vi "IMAQ Preview the image.vi"() -> ()   [LabVIEW 2018]
uses:
  LabViewDVPCamera/LabViewDVPCamera.lvlib
panel:
  in  "Video image quality (AVI format)":string
  in  "Recording Name (Path)":string
  in  "Turn on recording":bool
  out "Capture frame rate":sgl
  out "Total frame rate":u32
  out "pFrameCount out":T1
  out "frame rate":dbl format="%#.5g"
  out "value":u64
  out "Millisecond timing value 3":u32
  out "Image":T2(plugin-control)
  in  "CloseFlg":i32
  out "handle":u32
  in  "CameraList":u16(ring) items=["MGS130-H2-192.168.10.39", "MGS130-H2-192.168.10.4", "MGS203MP-H2-192.168.10.254", "MGS203MP-H2-192.168.20.2", "MGS230_YUV-H2-192.168.10.62"]
  in  "Set":bool
  in  "Close":bool
  in  "Open":bool
  in  "ScanCamera":bool
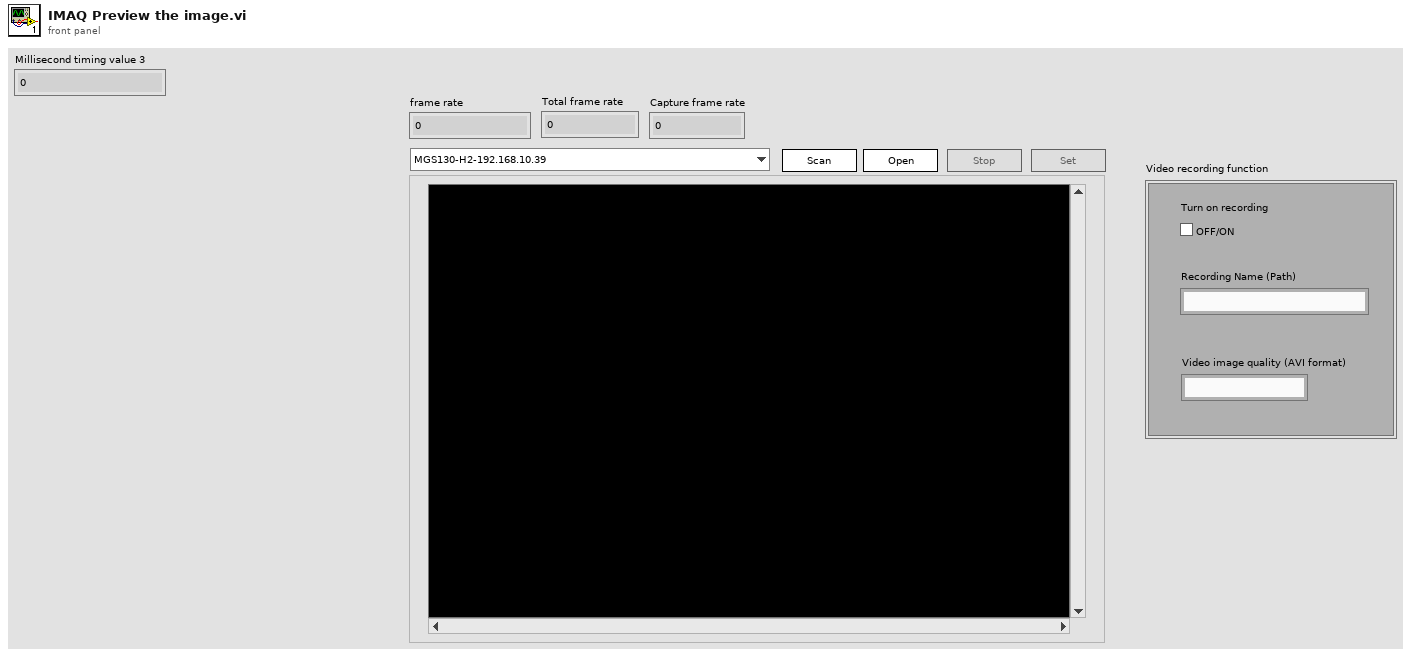
[diagram p1: front panel]
types:
  T1 = cluster{"uFrameCount":u32, "uFrameDrop":u32, "uFrameIgnore":u32, "uFrameError":u32, "uFrameOK":u32, "uFrameOut":u32, "uFrameResend":u32, "uFrameProc":u32, "fFrameRate":sgl, "fProcRate":sgl, "reserved[0]":i32, "reserved[1]":i32, "reserved[2]":i32, "reserved[3]":i32, "reserved[4]":i32, "reserved[5]":i32, "reserved[6]":i32, "reserved[7]":i32, "reserved[8]":i32, "reserved[9]":i32, "reserved[10]":i32, "reserved[11]":i32, "reserved[12]":i32, "reserved[13]":i32, "reserved[14]":i32, "reserved[15]":i32, "reserved[16]":i32, "reserved[17]":i32, "reserved[18]":i32, "reserved[19]":i32, "reserved[20]":i32, "reserved[21]":i32, "reserved[22]":i32, "reserved[23]":i32, "reserved[24]":i32, "reserved[25]":i32, "reserved[26]":i32, "reserved[27]":i32, "reserved[28]":i32, "reserved[29]":i32, "reserved[30]":i32, "reserved[31]":i32}
  T2 = typedef "IMAQ Image.ctl" = refnum<image>
  T3 = enum8{"Enabled", "Disabled", "Disabled and Grayed Out"}
  T4 = typedef "LVStringsAndValuesArrayTypeDef_U16.ctl" = cluster{"String":string, "Value":u16}[]
  T5 = typedef "Image Type" = u32
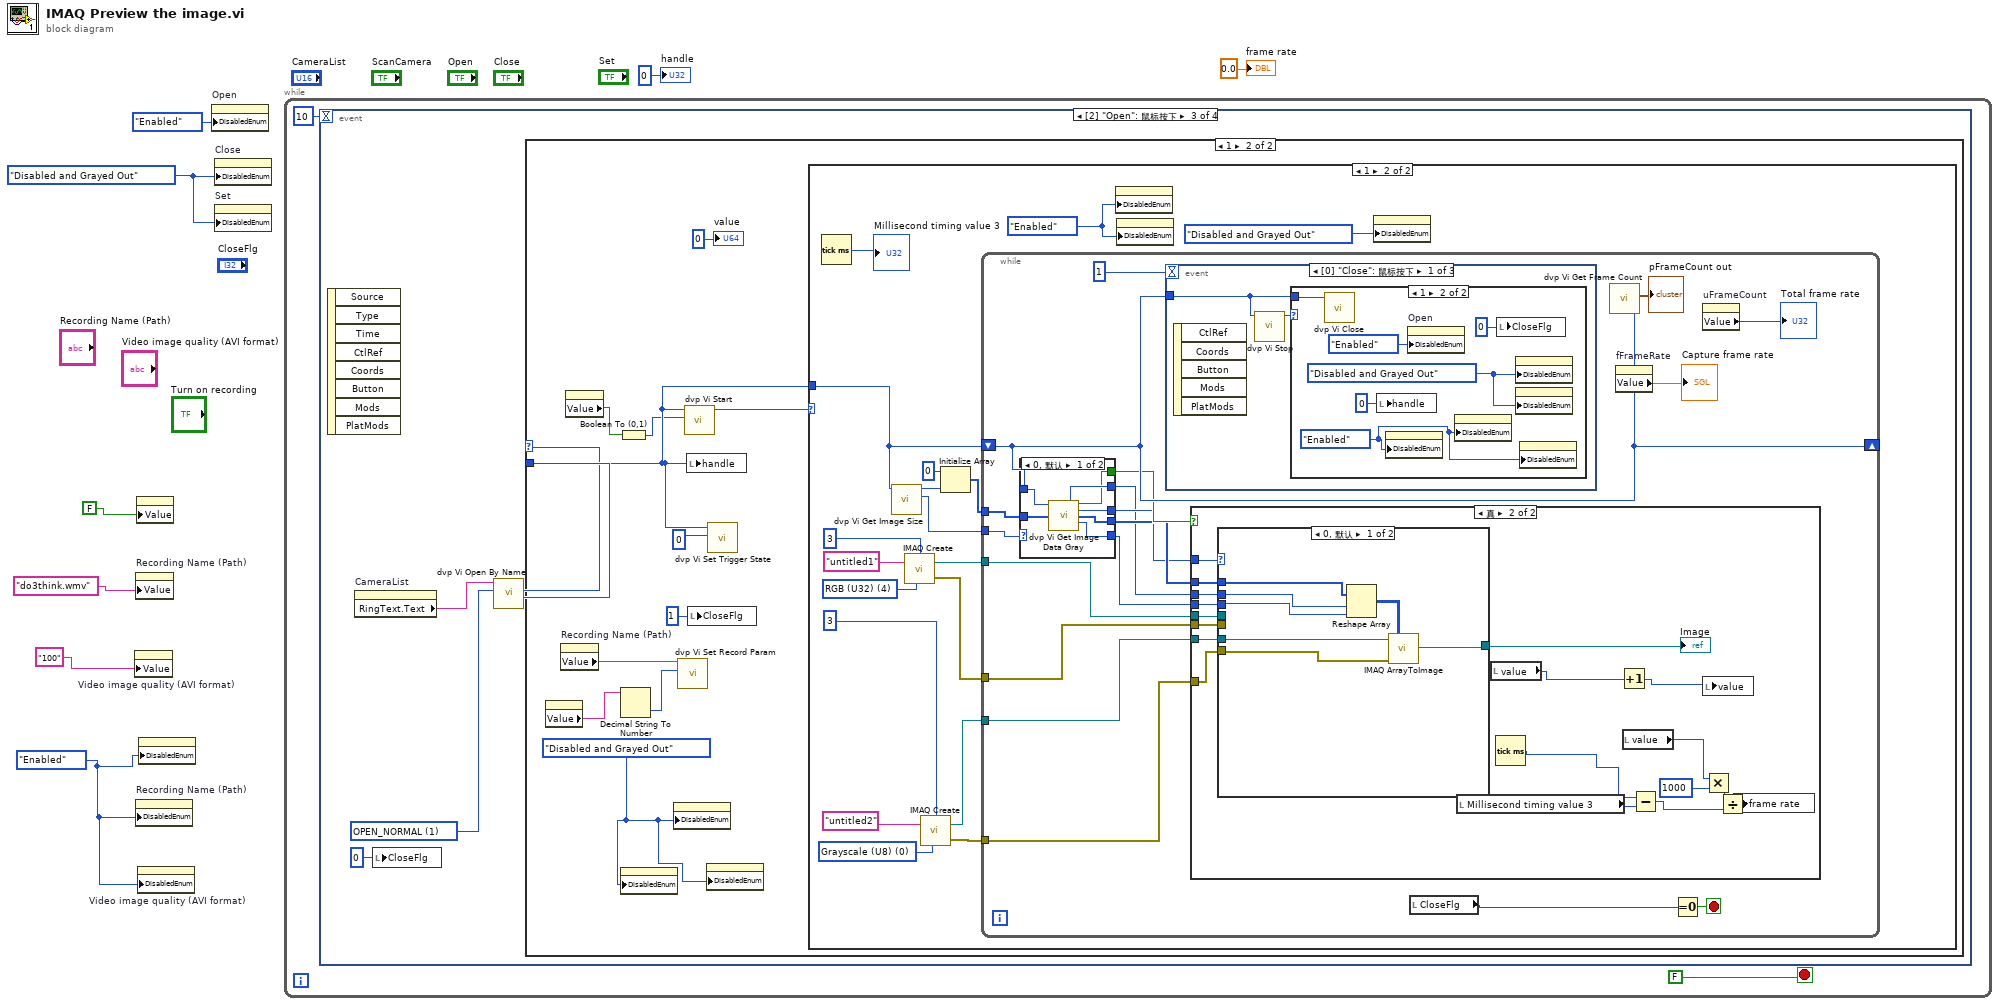
[diagram p0: block diagram]
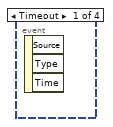
[diagram p2: hidden frame]
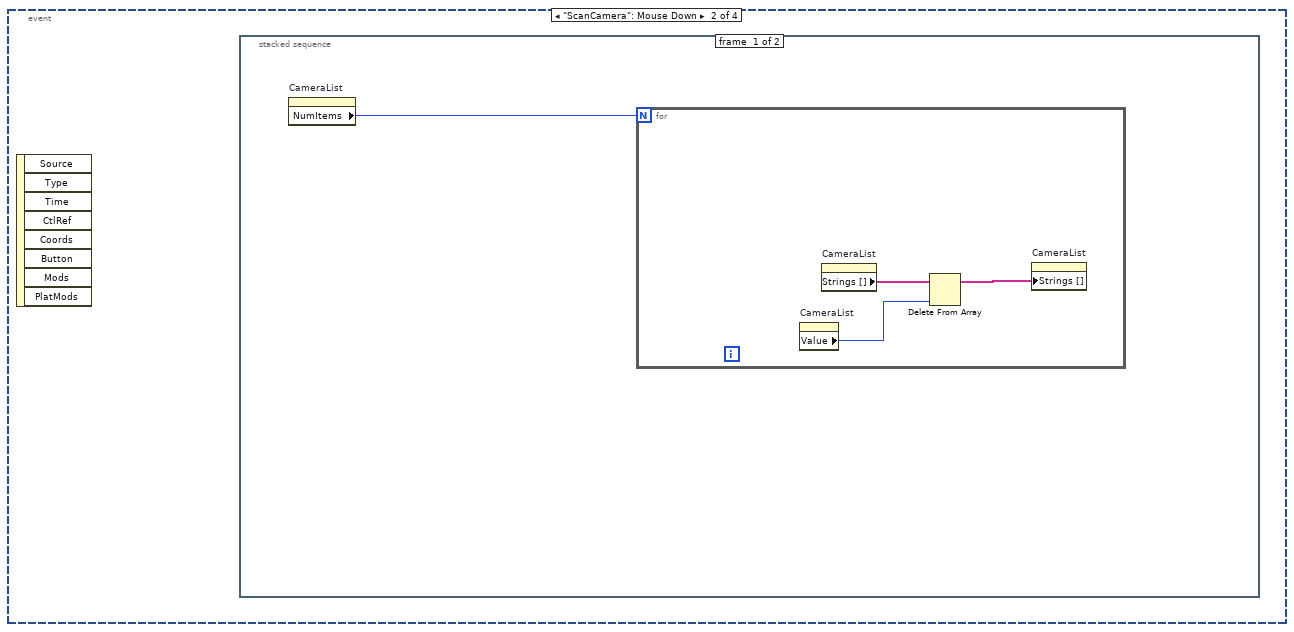
[diagram p3: hidden frame]
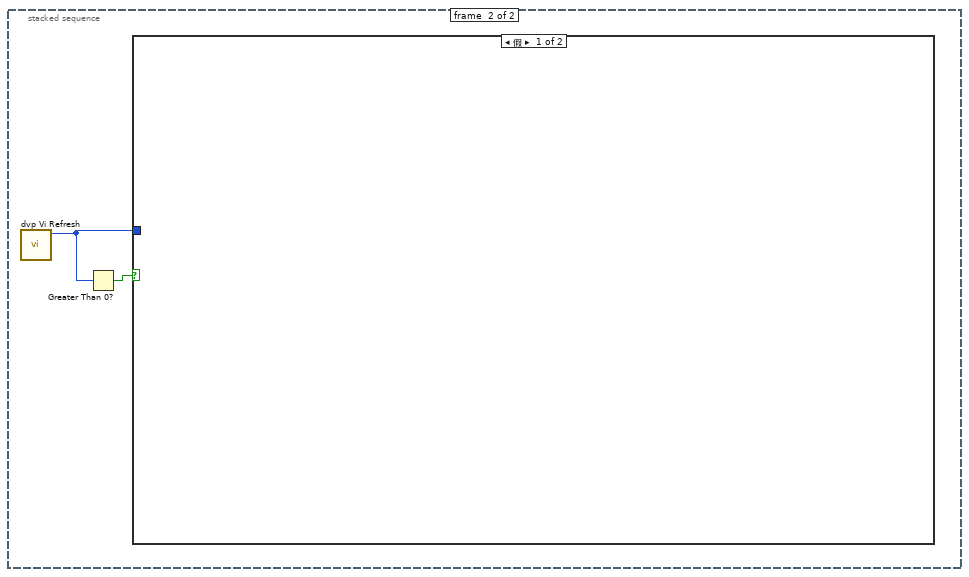
[diagram p4: hidden frame]
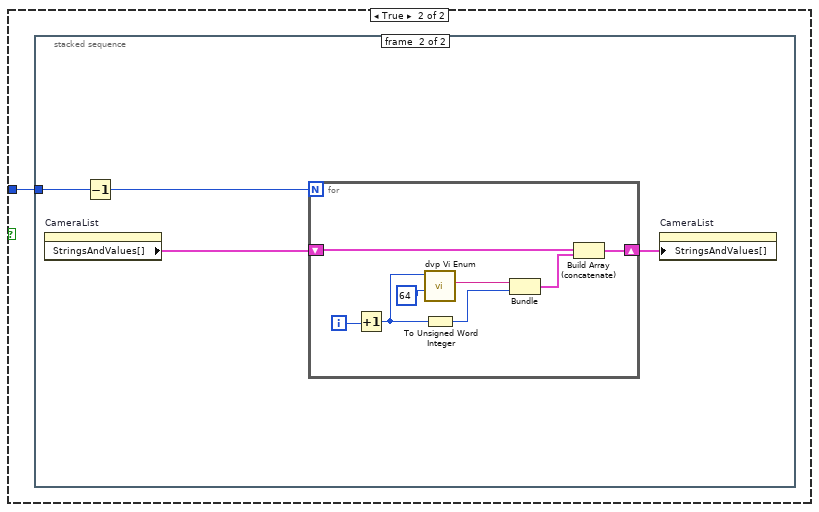
[diagram p5: hidden frame]
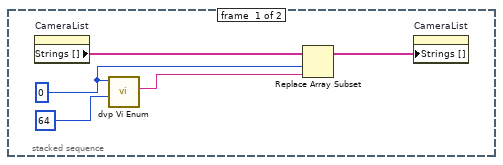
[diagram p6: hidden frame]
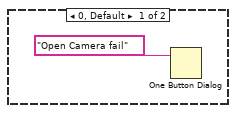
[diagram p7: hidden frame]
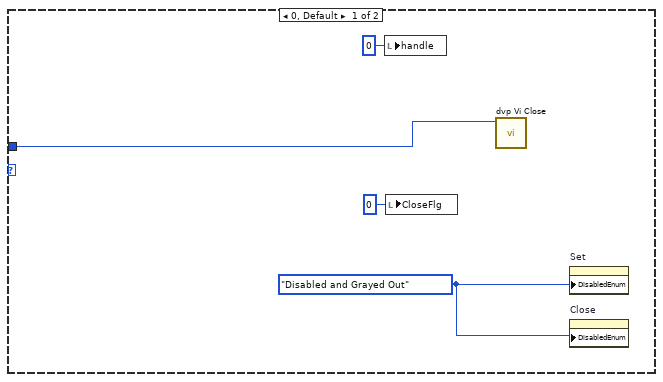
[diagram p8: hidden frame]
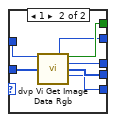
[diagram p9: hidden frame]
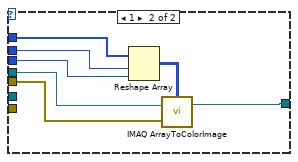
[diagram p11: hidden frame]
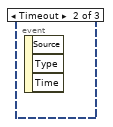
[diagram p13: hidden frame]
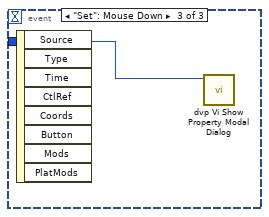
[diagram p14: hidden frame]
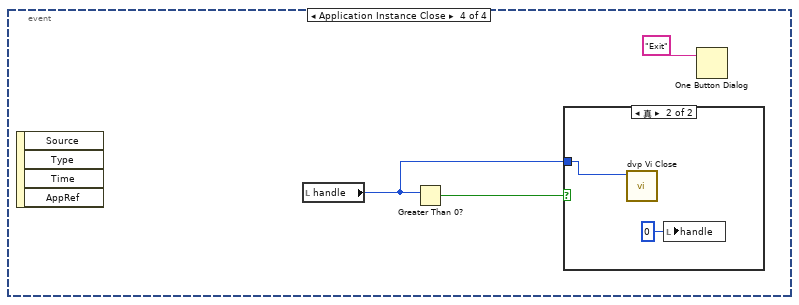
[diagram p15: hidden frame]
diagram:
  w1 = T3."Enabled" ("禁用")
  w7 = T3."Disabled and Grayed Out" ("禁用")
  n1 = property on="Video image quality (AVI format)" class="Str"("Value"="100") -> ()  [unwired: 2 in, 2 out]
  n2 = property on="Recording Name (Path)" class="Str"("Value"="do3think.wmv") -> ()  [unwired: 2 in, 2 out]
  n3 = property on="Recording Name (Path)" class="Str"("DisabledEnum"=w1) -> ()  [unwired: 2 in, 2 out]
  n4 = property class="Bool (严格)"("Value"=FALSE) -> ()  [unwired: 2 in, 2 out]
  n5 = property on="Video image quality (AVI format)" class="Str"("DisabledEnum"=w1) -> ()  [unwired: 2 in, 2 out]
  n6 = property class="Bool (严格)"("DisabledEnum"=w1) -> ()  [unwired: 2 in, 2 out]
  n7 = property on="Open" class="Bool"("DisabledEnum"=T3."Enabled" ("禁用")) -> ()  [unwired: 2 in, 2 out]
  n8 = property on="Close" class="Bool"("DisabledEnum"=w7) -> ()  [unwired: 2 in, 2 out]
  n9 = property on="Set" class="Bool"("DisabledEnum"=w7) -> ()  [unwired: 2 in, 2 out]
  n10 = while {
    stop <- FALSE stop-if-true
    n11 = event shown="[2] \"Open\": 鼠标按下" {
      selector: _ -> [_ _ _ _]
      dyn-events: _ -> [_ _ _ _]
      timeout: 10 -> [_ _ _ _]
      event Timeout {
        n12 = event-data() -> ()  [unwired: 1 in, 3 out]
      }
      event "ScanCamera": Mouse Down {
        n13 = event-data() -> ()  [unwired: 1 in, 8 out]
        n14 = stacked-sequence "清除下拉列表的数据" {
          frame #0 {
            n15 = property on="CameraList" class="Ring (严格)"() -> ("NumItems"=w11:u32)  [unwired: 2 in, 2 out]
            n16 = for {
              N: w11 -> [_]
              n17 = property on="CameraList" class="Ring (严格)"() -> ("Value"=w13:u16)  [unwired: 2 in, 2 out]
              n18 = property on="CameraList" class="Ring (严格)"() -> ("Strings []"=w12:string[])  [unwired: 2 in, 2 out]
              n19 = Delete From Array ("删除数组元素")(array=w12, index=w13) -> (array with subset deleted=w14:string[])  [unwired: 1 in, 1 out]
              n20 = property on="CameraList" class="Ring (严格)"("Strings []"=w14) -> ()  [unwired: 2 in, 2 out]
            }
          }
          frame #1 {
            n21 = call "dvp Vi Refresh.vi"() -> ("pCount out"=w16:u32)  [unwired: 10 in, 1 out]
            n22 = Greater Than 0?(x=w16) -> (x > 0?=w15:bool)
            n23 = case shown="假" w15 {
              tunnel: w16 -> [_ w17]
              frame False {
              }
              frame True {
                n24 = stacked-sequence {
                  tunnel: w17 -> [_ w24]
                  frame #0 {
                    w18 = u32 0 ("index")
                    n25 = property on="CameraList" class="Ring (严格)"() -> ("Strings []"=w21:string[])  [unwired: 2 in, 2 out]
                    n26 = call "dvp Vi Enum.vi"("unSize"=u32 64, "index"=w18) -> ("friendlyName out"=w20:string)  [unwired: 8 in, 1 out]
                    n27 = Replace Array Subset ("替换数组子集")(array=w21, new element=w20, index=w18) -> (w22:string[])
                    n28 = property on="CameraList" class="Ring (严格)"("Strings []"=w22) -> ()  [unwired: 2 in, 2 out]
                  }
                  frame #1 {
                    n29 = property on="CameraList" class="Ring (严格)"() -> ("StringsAndValues[]"=w26:T4)  [unwired: 2 in, 2 out]
                    n30 = Decrement(x=w24) -> (x-1=w23:u32)
                    n31 = for {
                      N: w23 -> [_]
                      shift-right: [w33] -> w25
                      shift-left: w26 -> [w31]
                      i -> [w28]
                      n32 = Increment(x=w28) -> (x+1=w27:i32)
                      n33 = call "dvp Vi Enum.vi"("unSize"=u32 64, "index"=w27) -> ("friendlyName out"=w34:string)  [unwired: 8 in, 1 out]
                      n34 = To Unsigned Word Integer(number=w27) -> (unsigned 16bit integer=w30:u16)
                      n35 = Bundle("friendlyName out"=w34, w30) -> (w32:cluster{"friendlyName out":string, u16})  [unwired: 1 in]
                      n36 = Build Array (concatenate) ("创建数组")(w31, w32) -> (w33:T4)
                    }
                    n37 = property on="CameraList" class="Ring (严格)"("StringsAndValues[]"=w25) -> ()  [unwired: 2 in, 2 out]
                  }
                }
              }
            }
          }
        }
      }
      event "Open": Mouse Down {
        w37 = u32 1 items=["OPEN_OFFLINE", "OPEN_NORMAL"] ("type")
        n38 = event-data() -> ()  [unwired: 1 in, 8 out]
        n39 = property on="CameraList" class="Ring (严格)"() -> ("RingText.Text"=w36:string)  [unwired: 2 in, 2 out]
        n40 = local write "CloseFlg"(0 ("CloseFlg")) -> ()
        n41 = call "dvp Vi Open By Name.vi"("type"=w37, "friendlyName"=w36) -> ("pHandle out"=w39:u32, "function return"=w38:u32)  [unwired: 7 in, 1 out]
        n42 = case shown="1" w38 {
          tunnel: w39 -> [_ w48]
          frame 0, Default {
            n43 = One Button Dialog(message="Open Camera fail" ("消息")) -> ()  [unwired: 1 in, 1 out]
          }
          frame 1 {
            w46 = T3."Disabled and Grayed Out" ("禁用")
            n44 = property class="Str"() -> ("Value"=w42:string)  [unwired: 2 in, 2 out]
            n45 = property on="Recording Name (Path)" class="Str"() -> ("Value"=w43:string)  [unwired: 2 in, 2 out]
            n46 = property class="Bool (严格)"() -> ("Value"=w45:bool)  [unwired: 2 in, 2 out]
            n47 = Boolean To (0,1)(Boolean=w45) -> (0, 1=w44:i16)
            n48 = Decimal String To Number(string=w42) -> (number=w41:i32)  [unwired: 2 in, 1 out]
            n49 = property class="Str"("DisabledEnum"=w46) -> ()  [unwired: 2 in, 2 out]
            n50 = property class="Bool (严格)"("DisabledEnum"=w46) -> ()  [unwired: 2 in, 2 out]
            n51 = call "dvp Vi Set Record Param.vi"("quality"=w41, "recordName"=w43) -> ()  [unwired: 8 in, 2 out]
            n52 = call "dvp Vi Start.vi"("bRecord"=w44, "handle"=w48) -> ("function return"=w50:u32)  [unwired: 9 in]
            n53 = local write "handle"(w48) -> ()
            n54 = local write "CloseFlg"(1 ("CloseFlg")) -> ()
            n55 = property class="Str"("DisabledEnum"=w46) -> ()  [unwired: 2 in, 2 out]
            n56 = call "dvp Vi Set Trigger State.vi"("TriggerState"=0, "handle"=w48) -> ()  [unwired: 9 in, 1 out]
            n57 = case shown="1" w50 {
              tunnel: w48 -> [w55 w69]
              frame 0, Default {
                w54 = T3."Disabled and Grayed Out" ("禁用")
                n58 = local write "handle"(u32 0 ("handle")) -> ()
                n59 = local write "CloseFlg"(0 ("CloseFlg")) -> ()
                n60 = call "dvp Vi Close.vi"("handle"=w55) -> ()  [unwired: 10 in, 1 out]
                n61 = property on="Set" class="Bool"("DisabledEnum"=w54) -> ()  [unwired: 2 in, 2 out]
                n62 = property on="Close" class="Bool"("DisabledEnum"=w54) -> ()  [unwired: 2 in, 2 out]
              }
              frame 1 {
                w64 = T5 4 items=["Grayscale (U8)", "Grayscale (I16)", "Grayscale (SGL)", "Complex (CSG)", "RGB (U32)", "HSL (U32)", "RGB (U64)", "Grayscale (U16)"] ("Image Type")
                w67 = T5 0 items=["Grayscale (U8)", "Grayscale (I16)", "Grayscale (SGL)", "Complex (CSG)", "RGB (U32)", "HSL (U32)", "RGB (U64)", "Grayscale (U16)"] ("Image Type")
                w73 = T3."Enabled" ("禁用")
                n63 = Tick Count (ms)() -> (millisecond timer value=→"Millisecond timing value 3":u32)
                n64 = call "dvp Vi Get Image Size.vi"("handle"=w69) -> ("pformat out"=w56:i32, "function return"=w68:u32)  [unwired: 9 in]
                n65 = call "IMAQ Create"("Border Size"=3, "Image Name"="untitled1", "Image Type"=w64) -> ("New Image"=w62:T2, "error out"=w61:errorcluster)  [unwired: 2 in]
                n66 = call "IMAQ Create"("Border Size"=3, "Image Name"="untitled2", "Image Type"=w67) -> ("New Image"=w59:T2, "error out"=w58:errorcluster)  [unwired: 2 in]
                n67 = Initialize Array(u8 0 ("元素"), w68) -> (w70:u8[])
                n68 = while {
                  shift-right: [w80] -> _
                  shift-left: w69 -> [w80]
                  tunnel: w70 -> [w81]
                  tunnel: w62 -> [w88]
                  tunnel: w61 -> [w87]
                  tunnel: w59 -> [w85]
                  tunnel: w58 -> [w86]
                  tunnel: w56 -> [w74]
                  stop <- w90 stop-if-true
                  n69 = case shown="0, 默认" w74 {
                    tunnel: w81 -> [w98 w105]
                    tunnel: w80 -> [w97 w104]
                    tunnel: [w93 w103] -> w79
                    tunnel: [w95 w102] -> w78
                    tunnel: [w94 w101] -> w77
                    tunnel: [w96 w100] -> w76
                    tunnel: [w92 w99] -> w75
                    frame 0, Default {
                      n70 = call "dvp Vi Get Image Data Gray.vi"("handle"=w97, "pbuffer"=w98) -> ("piHeight out"=w96:i32, "function return"=w93:bool, "pformat out"=w94:i32, "pbuffer out"=w95:u8[], "piWidth out"=w92:i32)  [unwired: 9 in]
                    }
                    frame 1 {
                      n71 = call "dvp Vi Get Image Data Rgb.vi"("handle"=w104, "pbuffer"=w105) -> ("piHeight out"=w100:i32, "function return"=w103:bool, "pformat out"=w101:i32, "pbuffer out"=w102:u32[], "piWidth out"=w99:i32)  [unwired: 9 in]
                    }
                  }
                  n72 = event shown="[0] \"Close\": 鼠标按下" {
                    selector: _ -> [_ _ _]
                    dyn-events: _ -> [_ _ _]
                    timeout: 1 -> [_ _ _]
                    tunnel: w80 -> [w138 _ w146]
                    event "Close": Mouse Down {
                      n73 = event-data() -> ()  [unwired: 1 in, 5 out]
                      n74 = call "dvp Vi Stop.vi"("handle"=w138) -> ("function return"=w139:u32)  [unwired: 10 in]
                      n75 = case shown="1" w139 {
                        tunnel: w138 -> [_ w143]
                        frame 0, Default {
                        }
                        frame 1 {
                          w140 = T3."Enabled" ("禁用")
                          w142 = T3."Disabled and Grayed Out" ("禁用")
                          n76 = call "dvp Vi Close.vi"("handle"=w143) -> ()  [unwired: 10 in, 1 out]
                          n77 = local write "handle"(u32 0 ("handle")) -> ()
                          n78 = property class="Bool (严格)"("DisabledEnum"=w140) -> ()  [unwired: 2 in, 2 out]
                          n79 = property on="Open" class="Bool"("DisabledEnum"=T3."Enabled" ("禁用")) -> ()  [unwired: 2 in, 2 out]
                          n80 = property class="Str"("DisabledEnum"=w140) -> ()  [unwired: 2 in, 2 out]
                          n81 = local write "CloseFlg"(0 ("CloseFlg")) -> ()
                          n82 = property on="Close" class="Bool"("DisabledEnum"=w142) -> ()  [unwired: 2 in, 2 out]
                          n83 = property on="Set" class="Bool"("DisabledEnum"=w142) -> ()  [unwired: 2 in, 2 out]
                          n84 = property class="Str"("DisabledEnum"=w140) -> ()  [unwired: 2 in, 2 out]
                        }
                      }
                    }
                    event Timeout {
                      n85 = event-data() -> ()  [unwired: 1 in, 3 out]
                    }
                    event "Set": Mouse Down {
                      n86 = event-data() -> ()  [unwired: 1 in, 8 out]
                      n87 = call "dvp Vi Show Property Modal Dialog.vi"("handle"=w146) -> ()  [unwired: 10 in, 1 out]
                    }
                  }
                  n88 = case shown="真" w79 {
                    tunnel: w75 -> [_ w123]
                    tunnel: w76 -> [_ w122]
                    tunnel: w78 -> [_ w120]
                    tunnel: w77 -> [_ w119]
                    tunnel: w88 -> [_ w117]
                    tunnel: w87 -> [_ w116]
                    tunnel: w86 -> [_ w115]
                    tunnel: w85 -> [_ w118]
                    frame False {
                    }
                    frame True {
                      n89 = case shown="0, 默认" w119 {
                        tunnel: w122 -> [w130 w136]
                        tunnel: w123 -> [w129 w137]
                        tunnel: [w128 w134] -> w121
                        tunnel: w120 -> [w124 w133]
                        tunnel: w118 -> [w125 _]
                        tunnel: w117 -> [_ w132]
                        tunnel: w116 -> [_ w131]
                        tunnel: w115 -> [w126 _]
                        frame 0, Default {
                          n90 = Reshape Array ("重排数组维数")(w124, w130, w129) -> (w127:u32[][])
                          n91 = call "IMAQ ArrayToImage"("error in (no error)"=w126, "Image Pixels (U8)"=w127, "Image"=w125) -> ("Image Out"=w128:T2)  [unwired: 7 in, 1 out]
                        }
                        frame 1 {
                          n92 = Reshape Array ("重排数组维数")(w133, w136, w137) -> (w135:u32[][])
                          n93 = call "IMAQ ArrayToColorImage"("Image Pixels (U32)"=w135, "Image"=w132, "error in (no error)"=w131) -> ("Image Out"=w134:T2)  [unwired: 2 in, 1 out]
                        }
                      }
                      "Image" <- w121
                      n94 = local read "Millisecond timing value 3"() -> (w112:u32)
                      n95 = local read "value"() -> (w109:u64)
                      n96 = Tick Count (ms)() -> (millisecond timer value=w111:u32)
                      n97 = Increment(x=w109) -> (x+1=w110:u64)
                      n98 = local read "value"() -> (w113:u64)
                      n99 = Subtract(x=w111, y=w112) -> (x-y=w106:u32)
                      n100 = local write "value"(w110) -> ()
                      n101 = Multiply(x=w113, y=u64 1000) -> (x*y=w108:u64)
                      n102 = Divide(x=w108, y=w106) -> (x/y=w114:dbl)
                      n103 = local write "frame rate"(w114) -> ()
                    }
                  }
                  n104 = local read "CloseFlg"() -> (w89:i32)
                  n105 = call "dvp Vi Get Frame Count.vi"("handle"=w80) -> ("pFrameCount out"=→"pFrameCount out":T1)  [unwired: 9 in, 1 out]
                  n106 = property on="fFrameRate" class="DigNum (严格)"() -> ("Value"=→"Capture frame rate":sgl)  [unwired: 2 in, 2 out]
                  n107 = Equal To 0?(x=w89) -> (x = 0?=w90:bool)
                  n108 = property on="uFrameCount" class="DigNum (严格)"() -> ("Value"=→"Total frame rate":u32)  [unwired: 2 in, 2 out]
                }
                n109 = property on="Set" class="Bool"("DisabledEnum"=w73) -> ()  [unwired: 2 in, 2 out]
                n110 = property on="Close" class="Bool"("DisabledEnum"=w73) -> ()  [unwired: 2 in, 2 out]
                n111 = property on="Open" class="Bool"("DisabledEnum"=T3."Disabled and Grayed Out" ("禁用")) -> ()  [unwired: 2 in, 2 out]
              }
            }
            "value" <- u64 0 ("数值")
          }
        }
      }
      event Application Instance Close {
        n112 = event-data() -> ()  [unwired: 1 in, 4 out]
        n113 = local read "handle"() -> (w147:u32)
        n114 = Greater Than 0?(x=w147) -> (x > 0?=w148:bool)
        n115 = case shown="真" w148 {
          tunnel: w147 -> [_ w151]
          frame False {
          }
          frame True {
            n116 = call "dvp Vi Close.vi"("handle"=w151) -> ()  [unwired: 10 in, 1 out]
            n117 = local write "handle"(u32 0 ("handle")) -> ()
          }
        }
        n118 = One Button Dialog(message="Exit" ("消息")) -> ()  [unwired: 1 in, 1 out]
      }
    }
  }
  "handle" <- u32 0 ("handle")
  "frame rate" <- 0.0 ("帧率")
